vi "固定站CODCr测量流程.vi"(11 "控制命令":T1(ring)) -> ()   [LabVIEW 2016, in "CODCr库.lvlib"]
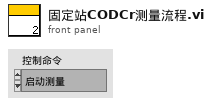
[diagram p1: front panel]
types:
  T1 = enum16{"启动测量", "标样核查", "零点核查", "跨度核查", "空白测试", "平行样测试", "加标回收", "空白校准", "标样校准", "初始化（清洗）", "停止测试", "仪器重启", "校时", "模式设置", "测量间隔设置"}
  T2 = cluster{"命令":string, "测量模式":enum16{"水样测量", "标样核查", "零点核查", "跨度核查", "空白测试", "加标回收", "平行样", "校零", "校标"}, "CODCr量程切换":enum32{"H", "L", "AUTO"}}
  T3 = cluster{"仪器":enum16{"", "氨氮", "总磷", "总氮", "CODMn", "CODCr"}, "启动命令":enum16{"启动水样流程", "启动加标流程", "排液", "停止", "柱塞泵启动"}}
  T4 = cluster{"时间标识":timestamp, "参数":string, "日志信息":string, "流程参数":string}
  T5 = enum16{"水样测量", "标样核查", "零点核查", "跨度核查", "空白测试", "加标回收", "平行样", "校零", "校标"}
  T6 = cluster{"命令":string, "测量模式":enum16{"水样测量", "标样核查", "零点核查", "跨度核查", "空白测试", "加标回收", "平行样", "校零", "校标"}, "CODMn量程切换":enum32{"H", "L", "AUTO"}}
  T7 = cluster{"系统时间":timestamp, "工作状态":u16, "测量模式":u16, "告警代码":u16, "故障代码":u16, "日志代码":u16, "软件版本":u16, "F0":sgl, "F1":sgl, "F2":sgl, "F3":sgl, "T":sgl, "H":sgl, "id":u16, "flowid":u16, "量程":u16}
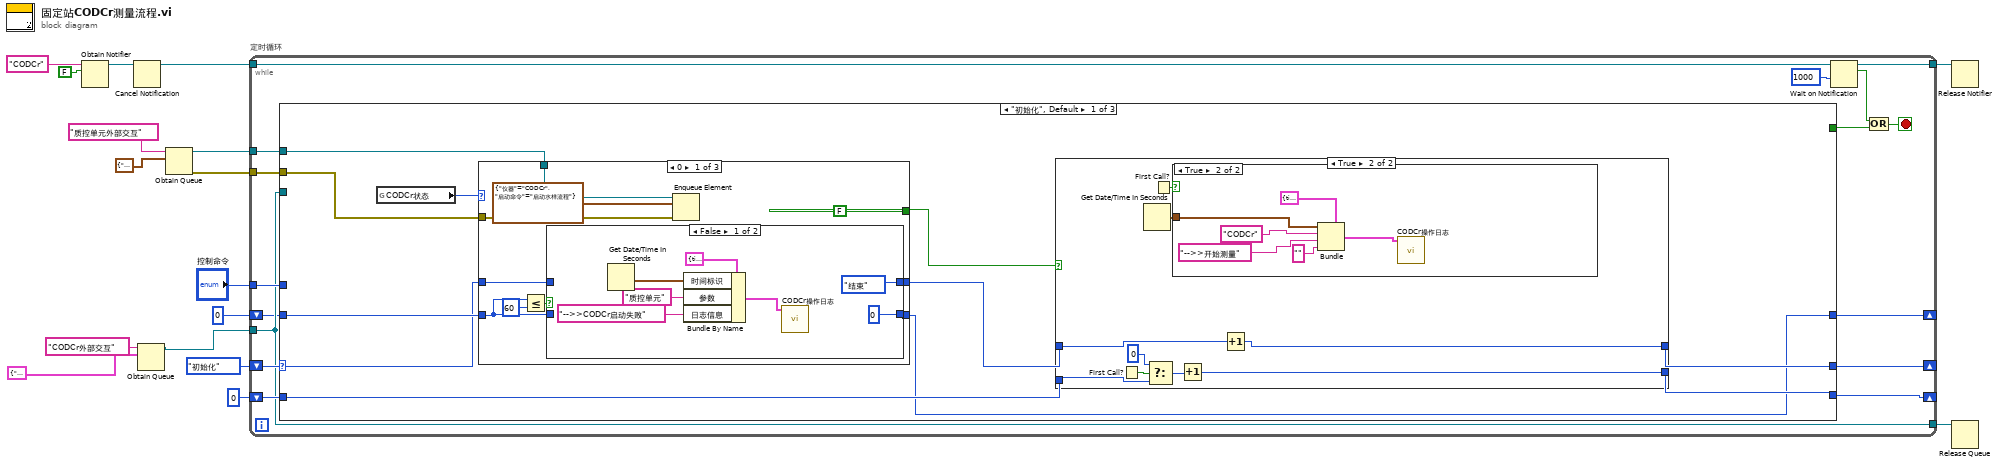
[diagram p0: block diagram]
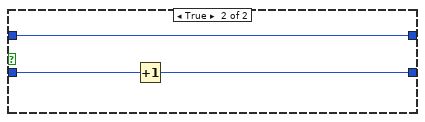
[diagram p4: hidden frame]
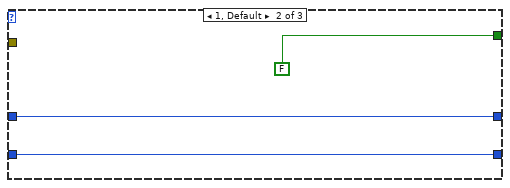
[diagram p5: hidden frame]
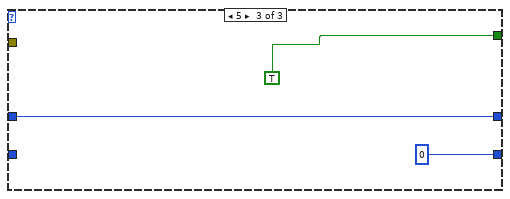
[diagram p6: hidden frame]
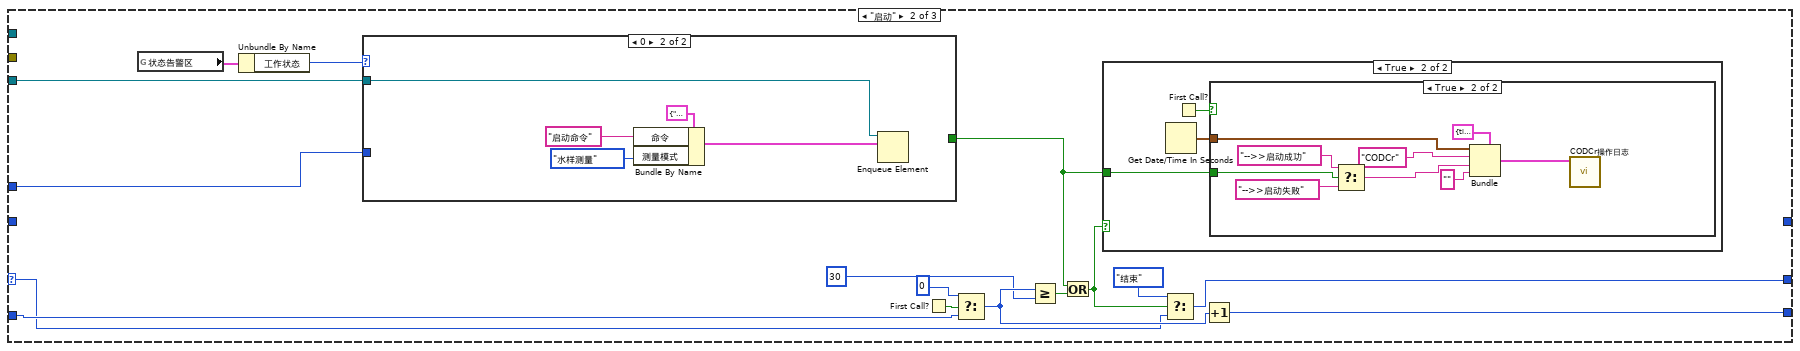
[diagram p7: hidden frame]
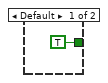
[diagram p10: hidden frame]
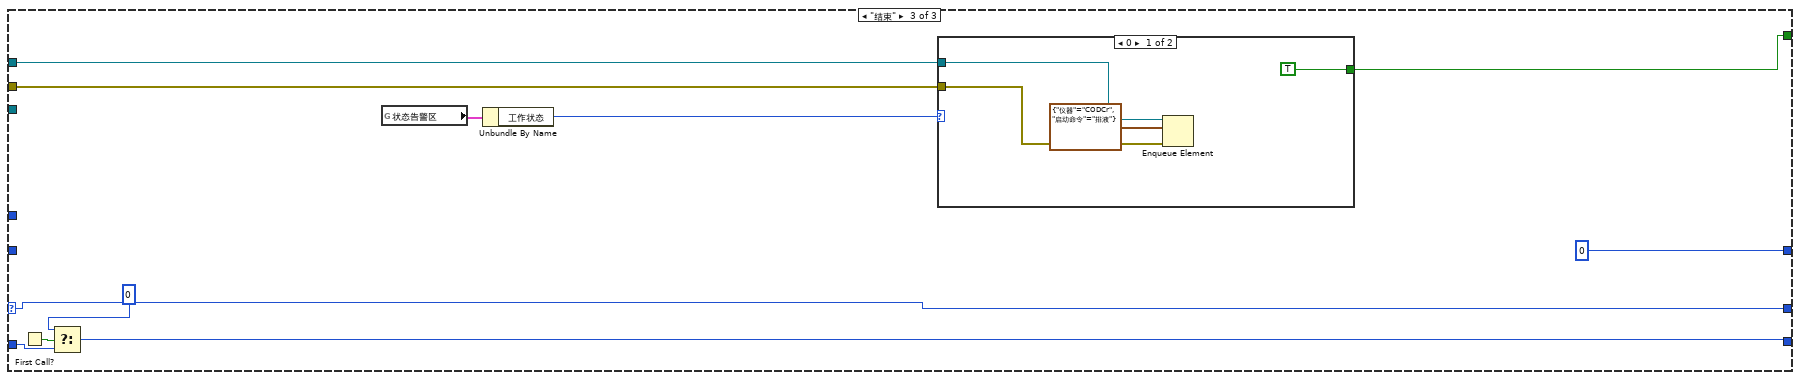
[diagram p11: hidden frame]
diagram:
  n1 = Obtain Notifier(name (unnamed)="CODCr" ("名称（未命名）"), notification data type=FALSE) -> (notifier out=w15:refnum<notifier>)  [unwired: 2 in, 2 out]
  n2 = Cancel Notification(0:w15) -> (8:w14:refnum<notifier>)  [unwired: 1 in, 2 out]
  n3 = Obtain Queue(name (unnamed)="CODCr外部交互" ("名称（未命名）"), element data type=T2 {"命令"="启动命令", "测量模式"=enum."水样测量", "CODCr量程切换"=enum."AUTO"} ("元素")) -> (queue out=w1:refnum<queue>)  [unwired: 3 in, 2 out]
  n4 = Obtain Queue(name (unnamed)="质控单元外部交互" ("名称（未命名）"), element data type=T3 {"仪器"=enum."氨氮", "启动命令"=enum."启动水样流程"} ("元素")) -> (queue out=w6:refnum<queue>, error out=w5:errorcluster)  [unwired: 3 in, 1 out]
  n5 = while "定时循环" {
    tunnel: w1 -> [w22]
    tunnel: w14 -> [w33]
    tunnel: "控制命令" -> [w28]
    shift-right: [w27] -> _
    shift-left: enum16{"初始化", "启动", "结束"}."初始化" -> [w29]
    shift-right: [w25] -> _
    shift-left: 0 -> [w26]
    tunnel: [w23] -> w10
    tunnel: [w22] -> w11
    tunnel: w6 -> [w21]
    tunnel: w5 -> [w20]
    shift-right: [w18] -> _
    shift-left: 0 -> [w19]
    stop <- w30 stop-if-true
    n6 = case shown="\"初始化\", Default" w29 {
      selector: w29 -> [w36 w94 w132]
      tunnel: w28 -> [_ w103 _]
      tunnel: w22 -> [_ w102 _]
      tunnel: [w44 w95 w132] -> w27
      tunnel: w26 -> [w43 w99 w129]
      tunnel: [w42 w98 w128] -> w25
      tunnel: [_ _ w125] -> w24
      tunnel: w21 -> [w40 _ w127]
      tunnel: w20 -> [w39 _ w126]
      tunnel: w19 -> [w38 _ _]
      tunnel: [w37 _ 0] -> w18
      frame "初始化", Default {
        n7 = global read "CODCr外部API.vi" "CODCr状态"() -> (w34:u16)
        n8 = case shown="0" w34 {
          tunnel: [FALSE ("s") FALSE ("s") TRUE ("s")] -> w41
          tunnel: w40 -> [w70 _ _]
          tunnel: w39 -> [w69 _ _]
          tunnel: w38 -> [w67 w82 _]
          tunnel: [w64 w82 0] -> w37
          tunnel: w36 -> [w63 w83 w86]
          tunnel: [w62 w83 w86] -> w35
          frame 0 {
            n9 = Less Or Equal?(x=w67, y=60) -> (x <= y?=w65:bool)
            n10 = case shown="False" w65 {
              tunnel: w67 -> [_ w81]
              tunnel: [0 w80] -> w64
              tunnel: w63 -> [_ w79]
              tunnel: [enum16{"初始化", "启动", "结束"}."结束" w79] -> w62
              frame False {
                n11 = Get Date/Time In Seconds() -> (seconds since 1Jan1904=w74:timestamp)
                n12 = Bundle By Name(cluster=T4 {"时间标识"=timestamp(0 s since 1904-01-01), "参数"="", "日志信息"="", "流程参数"=""} ("data in"), "时间标识"=w74, "参数"="质控单元" ("设备"), "日志信息"="-->>CODCr启动失败") -> (w72:T4)
                n13 = call "CODCr操作日志.vi"("data"=w72) -> ()  [unwired: 11 in]
              }
              frame True {
                n14 = Increment(x=w81) -> (x+1=w80:i32)
              }
            }
            n15 = Enqueue Element(queue=w70, element=T3 {"仪器"=enum."CODCr", "启动命令"=enum."启动水样流程"} ("元素"), error in (no error)=w69) -> ()  [unwired: 1 in, 3 out]
          }
          frame 1, Default {
          }
          frame 5 {
          }
        }
        n16 = case shown="True" w41 {
          tunnel: w35 -> [w46 w53]
          tunnel: [w46 w52] -> w44
          tunnel: w43 -> [w45 w50]
          tunnel: [w45 w47] -> w42
          frame False {
          }
          frame True {
            n17 = First Call?() -> (First Call?: T/F=w51:bool)
            n18 = Get Date/Time In Seconds() -> (seconds since 1Jan1904=w55:timestamp)
            n19 = Select(t=0, s=w51, f=w50) -> (s? t:f=w48:i32)
            n20 = First Call?() -> (First Call?: T/F=w54:bool)
            n21 = case shown="True" w54 {
              tunnel: w55 -> [_ w58]
              frame False {
              }
              frame True {
                n22 = Bundle(cluster=T4 {"时间标识"=timestamp(0 s since 1904-01-01), "参数"="", "日志信息"="", "流程参数"=""} ("data in"), "时间标识"=w58, "参数"="CODCr" ("设备"), "日志信息"="-->>开始测量", "流程参数"="" ("table输入")) -> (w56:T4)
                n23 = call "CODCr操作日志.vi"("data"=w56) -> ()  [unwired: 11 in]
              }
            }
            n24 = Increment(x=w48) -> (x+1=w47:i32)
            n25 = Increment(x=w53) -> (x+1=w52:enum16{"初始化", "启动", "结束"})
          }
        }
      }
      frame "启动" {
        n26 = global read "CODcr全局变量.vi" "状态告警区"() -> (w89:T7)
        n27 = Unbundle By Name(w89) -> ("工作状态"=w88:u16)
        n28 = case shown="0" w88 {
          tunnel: w103 -> [_ _]
          tunnel: w102 -> [_ w121]
          tunnel: [TRUE _] -> w90
          frame Default {
          }
          frame 0 {
            n29 = Bundle By Name(cluster=T6 {"命令"="启动命令", "测量模式"=enum."水样测量", "CODMn量程切换"=enum."AUTO"} ("元素"), "命令"="启动命令", "测量模式"=T5."水样测量") -> (w118:T6)
            n30 = Enqueue Element(queue=w121, element=w118) -> ()  [unwired: 2 in, 3 out]
          }
        }
        n31 = First Call?() -> (First Call?: T/F=w101:bool)
        n32 = Select(t=0, s=w101, f=w99) -> (s? t:f=w97:i32)
        n33 = Greater Or Equal?(x=w97, y=30) -> (x >= y?=w93:bool)
        n34 = Or(x=w90, y=w93) -> (x .or. y?=w91:bool)
        n35 = case shown="True" w91 {
          tunnel: w90 -> [_ w104]
          frame False {
          }
          frame True {
            n36 = Get Date/Time In Seconds() -> (seconds since 1Jan1904=w105:timestamp)
            n37 = First Call?() -> (First Call?: T/F=w106:bool)
            n38 = case shown="True" w106 {
              tunnel: w105 -> [_ w110]
              tunnel: w104 -> [_ w115]
              frame False {
              }
              frame True {
                n39 = Select(t="-->>启动成功" ("日志信息"), s=w115, f="-->>启动失败" ("日志信息")) -> (s? t:f=w108:string)
                n40 = Bundle(cluster=T4 {"时间标识"=timestamp(0 s since 1904-01-01), "参数"="", "日志信息"="", "流程参数"=""} ("data in"), "时间标识"=w110, "参数"="CODCr" ("设备"), "日志信息"=w108, "流程参数"="" ("table输入")) -> (w107:T4)
                n41 = call "CODCr操作日志.vi"("data"=w107) -> ()  [unwired: 11 in]
              }
            }
          }
        }
        n42 = Select(t=enum16{"初始化", "启动", "结束"}."结束", s=w91, f=w94) -> (s? t:f=w95:enum16{"初始化", "启动", "结束"})
        n43 = Increment(x=w97) -> (x+1=w98:i32)
      }
      frame "结束" {
        n44 = First Call?() -> (First Call?: T/F=w131:bool)
        n45 = Select(t=0, s=w131, f=w129) -> (s? t:f=w128:i32)
        n46 = global read "CODcr全局变量.vi" "状态告警区"() -> (w123:T7)
        n47 = Unbundle By Name(w123) -> ("工作状态"=w122:u16)
        n48 = case shown="0" w122 {
          tunnel: w127 -> [w135 _]
          tunnel: w126 -> [w134 _]
          tunnel: [TRUE _] -> w125
          frame 0 {
            n49 = Enqueue Element(queue=w135, element=T3 {"仪器"=enum."CODCr", "启动命令"=enum."排液"} ("元素"), error in (no error)=w134) -> ()  [unwired: 1 in, 3 out]
          }
          frame 1, Default {
          }
        }
      }
    }
    n50 = Wait on Notification(notifier=w33, timeout in ms (-1)=1000 ("超时毫秒(-1)")) -> (notifier out=w23:refnum<notifier>, notification=w31:bool)  [unwired: 2 in, 2 out]
    n51 = Or(x=w31, y=w24) -> (x .or. y?=w30:bool)
  }
  n52 = Release Notifier(notifier=w10) -> ()  [unwired: 2 in, 3 out]
  n53 = Release Queue(queue=w11) -> ()  [unwired: 2 in, 3 out]
